vi "WPI_CameraGet Frame Rate Notifier Internal.vi"(8 "error in (no error)":errorcluster, 11 "Camera Address":string) -> (0 "error out":errorcluster, 3 "Image Rate Notifier":refnum<notifier>)   [LabVIEW 2017]
doc: "This software is licensed. Open the labview\\readme\\WPI Robotics Library Open Source License.txt file for more information."
uses:
  <vilib>/Rock Robotics/WPI/Camera/WPI_CameraFrameRate.ctl
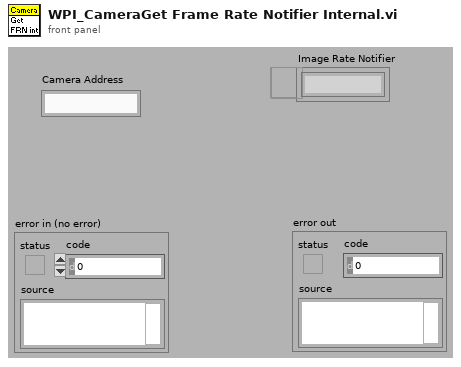
[diagram p1: front panel]
types:
  T1 = typedef "WPI_CameraFrameRate.ctl" = u32
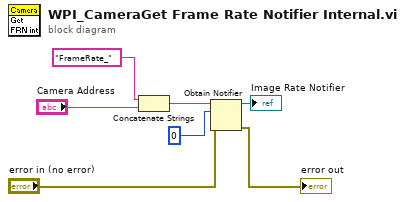
[diagram p0: block diagram]
diagram:
  n1 = Concatenate Strings("FrameRate_" ("format string"), "Camera Address") -> (w3:string)
  n2 = Obtain Notifier(name (unnamed)=w3, notification data type=T1 0 ("Frame Rate (fps)"), error in (no error)="error in (no error)") -> (notifier out=→"Image Rate Notifier":refnum<notifier>, error out=→"error out":errorcluster)  [unwired: 1 in, 1 out]
